vi "Singl_Qubit_Multpl.vi"(6 "Control Bitmask":bool[][](array[boolean]), 8 "error in (no error)":errorcluster, 9 "2x2 Unitary Matrix":cdb[][](array[numeric]), 10 "QuWire in":refnum<class "QuWire.lvclass">, 11 "QubitWiseMult in":refnum<class "QubitWiseMult.lvclass">) -> (0 "error out":errorcluster, 2 "QuWire out":refnum<class "QuWire.lvclass">, 3 "QubitWiseMult out":refnum<class "QubitWiseMult.lvclass">)   [LabVIEW 2020, in "QubitWiseMult.lvclass"]
uses:
  QubitWiseMult.lvclass
  QuWire/QuWire.lvclass
  QubitWiseMult.lvclass/QubitWiseMult.ctl
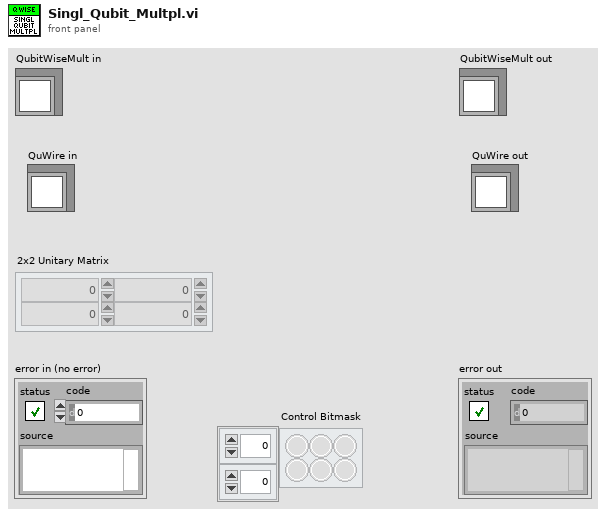
[diagram p1: front panel]
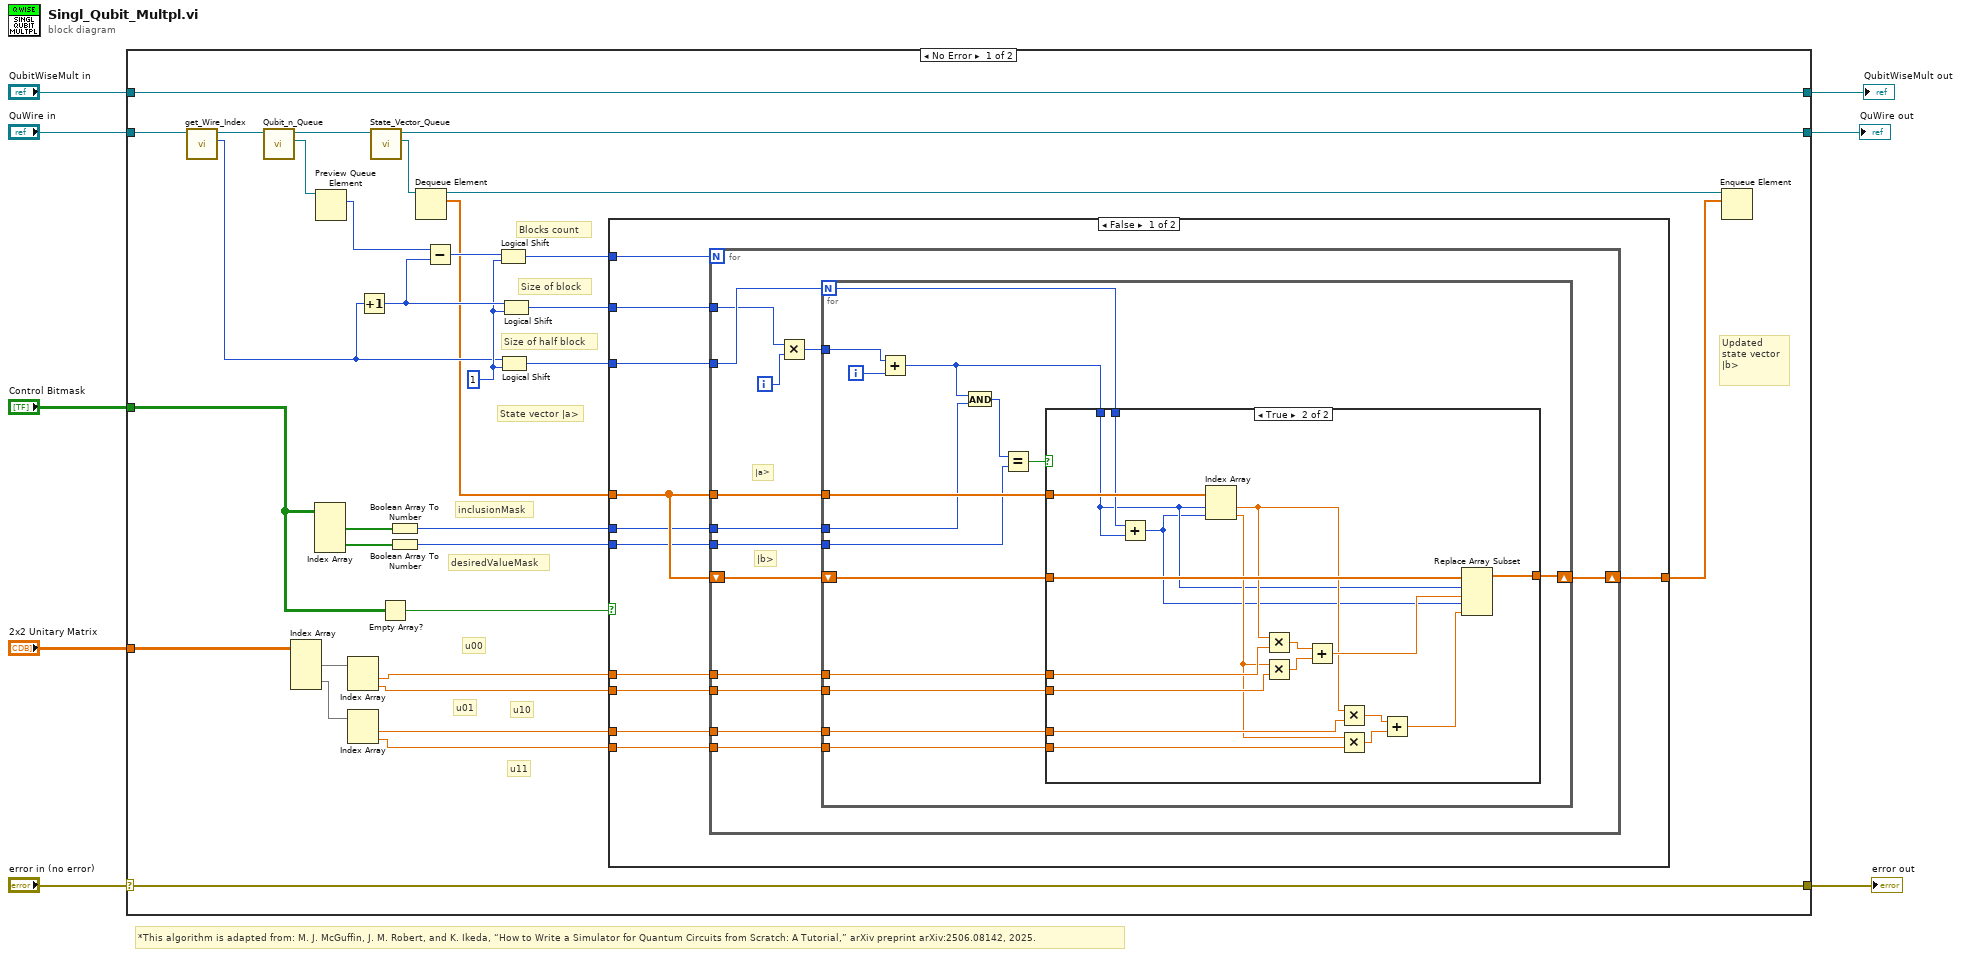
[diagram p0: block diagram]
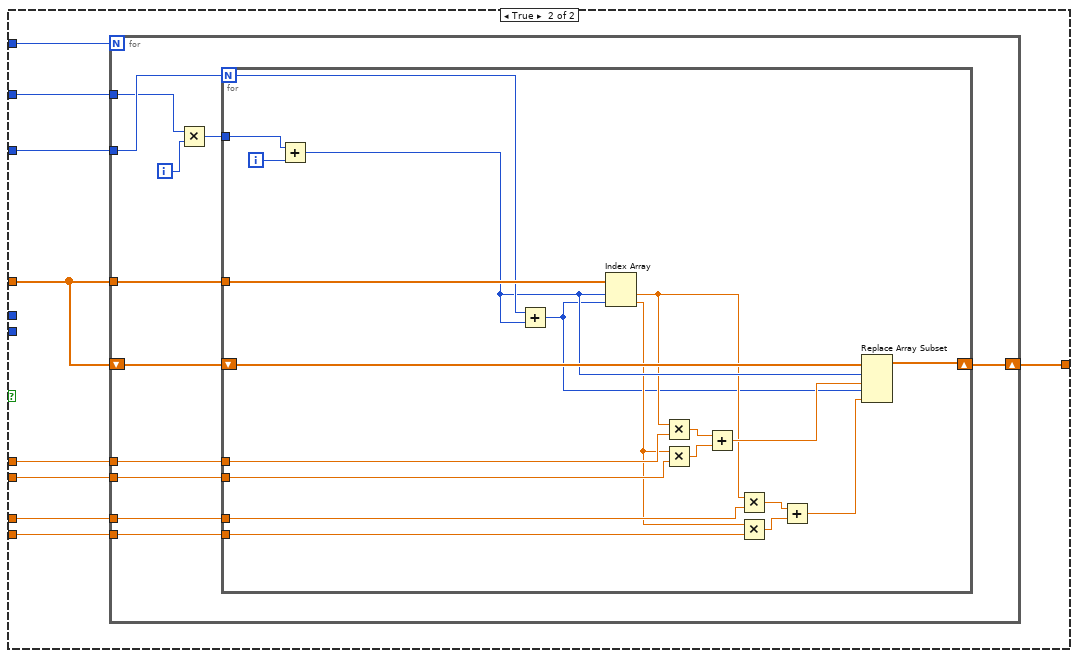
[diagram p3: hidden frame]
diagram:
  # "*This algorithm is adapted from: M. J. McGuffin, J. M. Robert, and K. Ikeda, “How to Write a Simulator for Quantum Circuits from Scratch: A Tutorial,” arXiv preprint arXiv:2506.08142, 2025."
  n1 = case shown="No Error" "error in (no error)" {
    selector: "error in (no error)" -> [w39 w141]
    tunnel: [w39 w141] -> w7
    tunnel: [w40 w140] -> w5
    tunnel: "QubitWiseMult in" -> [w40 w140]
    tunnel: "2x2 Unitary Matrix" -> [w13 _]
    tunnel: "Control Bitmask" -> [w12 _]
    tunnel: "QuWire in" -> [w11 w139]
    tunnel: [w10 w139] -> w1
    frame No Error {
      w34 = 1 ("x")
      # "Updated state vector |b>"
      # "State vector |a>"
      # "u11"
      # "u10"
      # "u01"
      # "u00"
      # "inclusionMask"
      # "desiredValueMask"
      # "Blocks count"
      # "Size of block"
      # "Size of half block"
      n2 = call "get_Wire_Index.vi"("QuWire in"=w11) -> ("Wire Index"=w33:i32, "QuWire out"=w23:refnum<class "QuWire.lvclass">)  [unwired: 8 in, 1 out]
      n3 = call "Qubit_n_Queue.vi"("QuWire in"=w23) -> ("Qubit n"=w24:refnum<queue>, "QuWire out"=w25:refnum<class "QuWire.lvclass">)  [unwired: 8 in, 1 out]
      n4 = Index Array(array=w13) -> (element #1=w18:cdb[], element #2=w19:cdb[])  [unwired: 4 in]
      n5 = Index Array(array=w12) -> (element #1=w22:bool[], element #2=w21:bool[])  [unwired: 4 in]
      n6 = Preview Queue Element(queue=w24) -> (element=w36:i32)  [unwired: 2 in, 3 out]
      n7 = Index Array(array=w18) -> (element #1=w17:cdb, element #2=w16:cdb)  [unwired: 2 in]
      n8 = Index Array(array=w19) -> (element #1=w9:cdb, element #2=w14:cdb)  [unwired: 2 in]
      n9 = Increment(x=w33) -> (x+1=w37:i32)
      n10 = call "State_Vector_Queue.vi"("QuWire in"=w25) -> ("State Vector Queue"=w26:refnum<queue>, "QuWire out"=w10:refnum<class "QuWire.lvclass">)  [unwired: 8 in, 1 out]
      n11 = Empty Array?(array=w12) -> (empty?=w31:bool)
      n12 = Boolean Array To Number(Boolean array=w22) -> (number=w20:u32)
      n13 = Boolean Array To Number(Boolean array=w21) -> (number=w30:u32)
      n14 = Dequeue Element(queue=w26) -> (queue out=w28:refnum<queue>, element=w27:cdb[])  [unwired: 2 in, 2 out]
      n15 = Subtract(x=w36, y=w37) -> (x-y=w38:i32)
      n16 = Logical Shift(y=w38, x=w34) -> (x << y=w32:i32)
      n17 = Logical Shift(y=w33, x=w34) -> (x << y=w15:i32)
      n18 = Logical Shift(y=w37, x=w34) -> (x << y=w35:i32)
      n19 = case shown="False" w31 {
        tunnel: w14 -> [w42 w100]
        tunnel: w9 -> [w43 w101]
        tunnel: w15 -> [w49 w105]
        tunnel: w16 -> [w44 w102]
        tunnel: w17 -> [w45 w103]
        tunnel: w30 -> [w46 _]
        tunnel: w20 -> [w47 _]
        tunnel: w27 -> [w48 w104]
        tunnel: [w41 w99] -> w29
        tunnel: w32 -> [w51 w107]
        tunnel: w35 -> [w50 w106]
        frame False {
          n20 = for {
            N: w51 -> [_]
            tunnel: w48 -> [w64]
            tunnel: w50 -> [w59]
            shift-right: [w63] -> w41
            shift-left: w48 -> [w62]
            tunnel: w49 -> [w61]
            tunnel: w45 -> [w57]
            tunnel: w44 -> [w56]
            tunnel: w43 -> [w55]
            tunnel: w42 -> [w54]
            tunnel: w47 -> [w53]
            tunnel: w46 -> [w52]
            i -> [w60]
            # "|a>"
            # "|b>"
            n21 = Multiply(x=w59, y=w60) -> (x*y=w58:i32)
            n22 = for {
              N: w61 -> [w76]
              tunnel: w64 -> [w79]
              shift-right: [w78] -> w63
              shift-left: w62 -> [w77]
              tunnel: w58 -> [w74]
              tunnel: w57 -> [w73]
              tunnel: w56 -> [w72]
              tunnel: w55 -> [w71]
              tunnel: w54 -> [w70]
              tunnel: w53 -> [w66]
              tunnel: w52 -> [w65]
              i -> [w75]
              n23 = Add(x=w74, y=w75) -> (x+y=w69:i32)
              n24 = And(x=w69, y=w66) -> (x .and. y?=w68:u32)
              n25 = Equal?(x=w68, y=w65) -> (x = y?=w67:bool)
              n26 = case shown="True" w67 {
                tunnel: w79 -> [_ w98]
                tunnel: [w80 w97] -> w78
                tunnel: w77 -> [w80 w96]
                tunnel: w76 -> [_ w95]
                tunnel: w73 -> [_ w94]
                tunnel: w72 -> [_ w92]
                tunnel: w71 -> [_ w87]
                tunnel: w70 -> [_ w86]
                tunnel: w69 -> [_ w82]
                frame False {
                }
                frame True {
                  n27 = Add(x=w95, y=w82) -> (x+y=w81:i32)
                  n28 = Index Array(array=w98, index #1=w82, index #2=w81) -> (element #1=w85:cdb, element #2=w84:cdb)
                  n29 = Multiply(x=w85, y=w94) -> (x*y=w93:cdb)
                  n30 = Multiply(x=w84, y=w92) -> (x*y=w91:cdb)
                  n31 = Add(x=w93, y=w91) -> (x+y=w90:cdb)
                  n32 = Multiply(x=w85, y=w87) -> (x*y=w88:cdb)
                  n33 = Multiply(x=w84, y=w86) -> (x*y=w89:cdb)
                  n34 = Add(x=w88, y=w89) -> (x+y=w83:cdb)
                  n35 = Replace Array Subset(array=w96, new element #1=w90, index #1=w82, new element #2=w83, index #2=w81) -> (w97:cdb[])
                }
              }
            }
          }
        }
        frame True {
          n36 = for {
            N: w107 -> [_]
            tunnel: w104 -> [w118]
            tunnel: w106 -> [w113]
            shift-right: [w117] -> w99
            shift-left: w104 -> [w116]
            tunnel: w105 -> [w115]
            tunnel: w103 -> [w111]
            tunnel: w102 -> [w110]
            tunnel: w101 -> [w109]
            tunnel: w100 -> [w108]
            i -> [w114]
            n37 = Multiply(x=w113, y=w114) -> (x*y=w112:i32)
            n38 = for {
              N: w115 -> [w135]
              tunnel: w118 -> [w138]
              shift-right: [w137] -> w117
              shift-left: w116 -> [w136]
              tunnel: w112 -> [w133]
              tunnel: w111 -> [w132]
              tunnel: w110 -> [w131]
              tunnel: w109 -> [w130]
              tunnel: w108 -> [w129]
              i -> [w134]
              n39 = Add(x=w133, y=w134) -> (x+y=w128:i32)
              n40 = Add(x=w135, y=w128) -> (x+y=w119:i32)
              n41 = Index Array(array=w138, index #1=w128, index #2=w119) -> (element #1=w122:cdb, element #2=w121:cdb)
              n42 = Multiply(x=w122, y=w132) -> (x*y=w127:cdb)
              n43 = Multiply(x=w121, y=w131) -> (x*y=w126:cdb)
              n44 = Add(x=w127, y=w126) -> (x+y=w125:cdb)
              n45 = Multiply(x=w122, y=w130) -> (x*y=w123:cdb)
              n46 = Multiply(x=w121, y=w129) -> (x*y=w124:cdb)
              n47 = Add(x=w123, y=w124) -> (x+y=w120:cdb)
              n48 = Replace Array Subset(array=w136, new element #1=w125, index #1=w128, new element #2=w120, index #2=w119) -> (w137:cdb[])
            }
          }
        }
      }
      n49 = Enqueue Element(queue=w28, element=w29) -> ()  [unwired: 2 in, 3 out]
    }
    frame Error {
    }
  }
  "error out" <- w7
  "QubitWiseMult out" <- w5
  "QuWire out" <- w1
